vi "jiffy_QuitarComillas.vi"(1 "String in":string) -> (0 "String out":string)   [LabVIEW 2017]
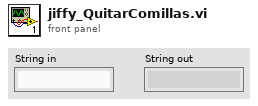
[diagram p1: front panel]
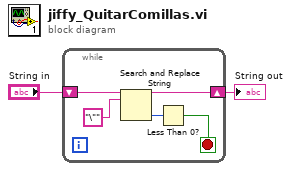
[diagram p0: block diagram]
diagram:
  n1 = while {
    shift-right: [w5] -> w2
    shift-left: "String in" -> [w7]
    stop <- w3 stop-if-true
    n2 = Search and Replace String(input string=w7, search string="\"") -> (result string=w5:string, offset past replacement=w4:i32)  [unwired: 6 in, 2 out]
    n3 = Less Than 0?(x=w4) -> (x < 0?=w3:bool)
  }
  "String out" <- w2
